vi "PID Set Contraints.vi"(9 "Profiled Contraints":T1, 10 "Output Range":cluster{"output high":dbl, "output low":dbl}, 11 "PID Ref":refnum<data-value>) -> (3 "PID Ref":refnum<data-value>)   [LabVIEW 2019]
uses:
  Typedef/PID Controller State.ctl
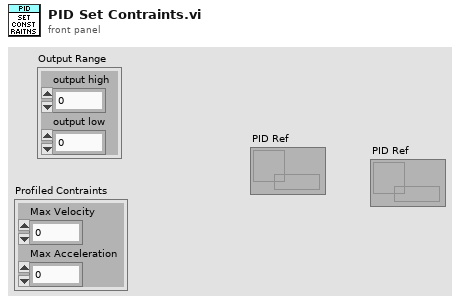
[diagram p1: front panel]
types:
  T1 = cluster{"Max Velocity":dbl, "Max Acceleration":dbl}
  T2 = typedef "PID Controller State.ctl" = cluster{"PIDF Gains":cluster{"Kp":dbl, "Ki":dbl, "Kd":dbl, "Kf":dbl}, "Output Range":cluster{"output high":dbl, "output low":dbl}, "Profiled?":bool, "PID State":cluster{"iState":dbl, "dState":dbl, "Error [n-1]":dbl, "Output":dbl}, "Setpoint":dbl, "Profiled State":cluster{"Position":dbl, "Velocity":dbl}, "Profiled Contraints":cluster{"Max Velocity":dbl, "Max Acceleration":dbl}}
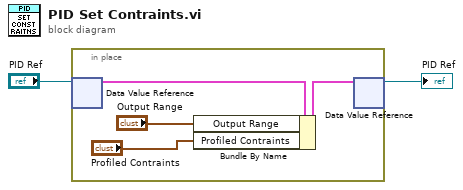
[diagram p0: block diagram]
diagram:
  n1 = in-place {
    n2 = in-place-dvr #1("PID Ref") -> (w6:T2)  [unwired: 1 out]
    n3 = Bundle By Name(cluster=w6, "Output Range"="Output Range", "Profiled Contraints"="Profiled Contraints") -> (w5:T2)
    n4 = in-place-dvr #1(w5) -> (→"PID Ref":refnum<data-value>)  [unwired: 1 out]
  }
